vi "Destroy Embedded Progress Bar.vi"(8 "Error In":errorcluster, 11 "Progress Bar Queue in":refnum<queue>) -> (0 "Error Out":errorcluster)   [LabVIEW 2021, in "GUI.lvlib"]
uses:
  GUI.lvlib
  Embedded Progress Bar Q Element.ctl
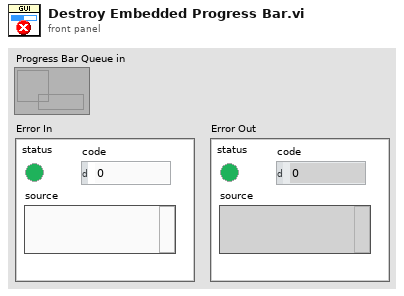
[diagram p1: front panel]
types:
  T1 = typedef "GUI.lvlib/Embedded Progress Bar Q Element.ctl" = cluster{"Action":string, "Value":dbl}
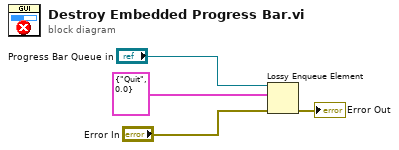
[diagram p0: block diagram]
diagram:
  n1 = Lossy Enqueue Element(queue="Progress Bar Queue in", element=T1 {"Action"="Quit", "Value"=0.0}, error in (no error)="Error In") -> (error out=→"Error Out":errorcluster)  [unwired: 3 out]
